vi "TxChannel - Create Channel Configuration.vi"(8 "error in (no error)":errorcluster, 11 "Parent Packet Ref":T1 format="%.0x") -> (0 "error out":errorcluster, 2 "Channel Config Ref":T1 format="%.0x")   [LabVIEW 2016, in "UDP-Custom-Device System Explorer.lvlib"]
uses:
  UDP-Custom-Device System Explorer.lvlib
  <vilib>/NI Veristand/Custom Device API/Custom Device Item Ref.ctl
  <vilib>/NI Veristand/Custom Device API/Custom Device Channel.ctl
  <vilib>/NI Veristand/Custom Device API/Custom Device Channel Type.ctl
  Shared/Constants.vi
  <vilib>/NI VeriStand/Custom Device API/Custom Device API.lvlib
  Shared/UDP-Custom-Device Shared.lvlib
  Property Accessors/Shared Channel Accessors.lvlib
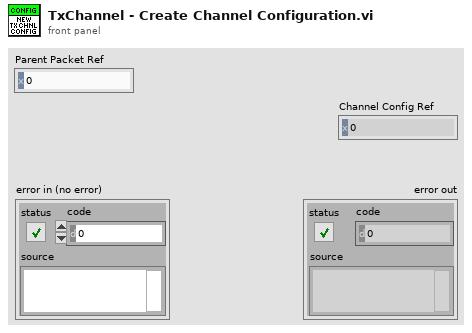
[diagram p1: front panel]
types:
  T1 = typedef "Custom Device API.lvlib/Custom Device Item Ref.ctl" = u64
  T2 = typedef "Custom Device API.lvlib/Custom Device Channel.ctl" = cluster{"Type":T3, "Units":string, "Default Value":dbl, "Faultable":bool, "Scalable":bool}
  T3 = typedef "Custom Device API.lvlib/Custom Device Channel Type.ctl" = enum16{"Input", "Output"}
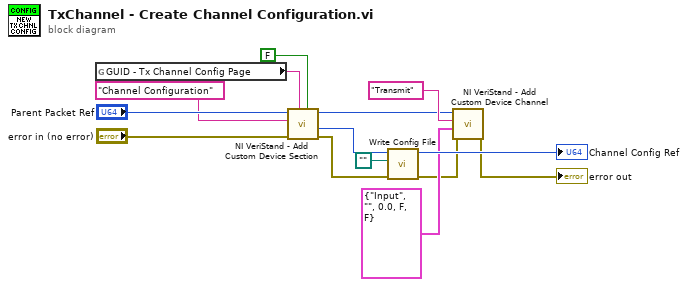
[diagram p0: block diagram]
diagram:
  n1 = global read "Constants.vi" "GUID - Tx Channel Config Page"() -> (w11:string)
  n2 = call <vilib>:"NI VeriStand - Add Custom Device Section.vi"("Highlight? (F)"=FALSE, "GUID (Default Section)"=w11, "error in (no error)"="error in (no error)", "Section Name"="Channel Configuration", "Parent Ref in"="Parent Packet Ref") -> ("error out"=w6:errorcluster, "Section Ptr"=w7:T1, "Parent Ref out"=w3:T1)  [unwired: 3 in, 1 out]
  n3 = call "Write Config File.vi"("error in (no error)"=w6, "Config File"=path "", "Node Ptr"=w7) -> ("error out"=w2:errorcluster, "Node Ptr out"=→"Channel Config Ref":T1)  [unwired: 7 in]
  n4 = call <vilib>:"NI VeriStand - Add Custom Device Channel.vi"("error in (no error)"=w2, "Channel"=T2 {"Type"=enum."Input", "Units"="", "Default Value"=0.0, "Faultable"=FALSE, "Scalable"=FALSE}, "Channel Name"="Transmit", "Parent Ref in"=w3) -> ("error out"=→"error out":errorcluster)  [unwired: 4 in, 3 out]
